vi "getImage.vi"(4 "Streeam":bool, 5 "imageError IN":errorcluster, 6 "Image IN":T1, 7 "errorCamera IN":errorcluster, 8 "hCamera IN":u32) -> (0 "errorImage OUT":errorcluster, 1 "Image OUT":T1, 2 "errorCamera OUT":errorcluster, 3 "hCamera OUT":u32)   [LabVIEW 2010]
uses:
  <vilib>/vision/Image Controls.llb/IMAQ Image.ctl
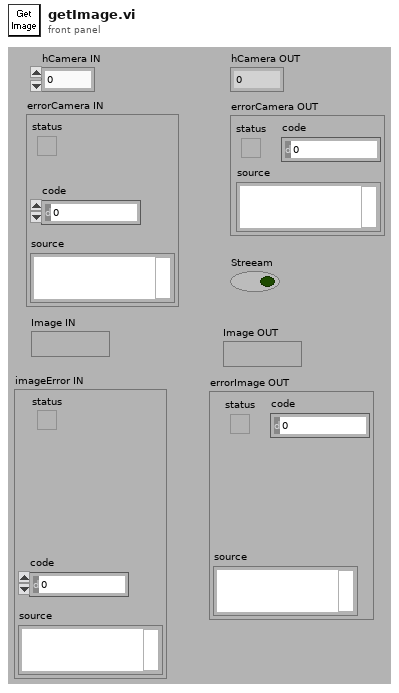
[diagram p1: front panel]
types:
  T1 = typedef "IMAQ Image.ctl" = refnum<image>
  T2 = enum32{"Map Pixel Pointer", "Unmap Pixel Pointer", "Get Pixels Infos"}
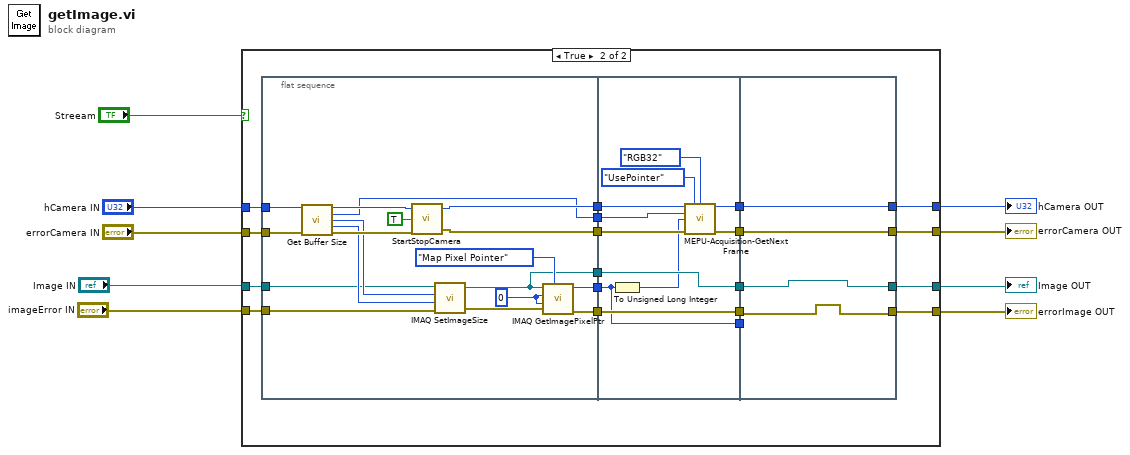
[diagram p0: block diagram]
diagram:
  n1 = case shown="True" "Streeam" {
    tunnel: "hCamera IN" -> [w13 w27]
    tunnel: "errorCamera IN" -> [w12 w26]
    tunnel: "Image IN" -> [w11 w25]
    tunnel: "imageError IN" -> [w10 w24]
    tunnel: [w11 w23] -> w4
    tunnel: [w10 w22] -> w3
    tunnel: [w12 w21] -> w2
    tunnel: [w13 w20] -> w1
    frame False {
    }
    frame True {
      n2 = flat-sequence {
        tunnel: [w48] -> w32
        tunnel: [w47] -> w31
        tunnel: w25 -> [w44]
        tunnel: w24 -> [w43]
        tunnel: w27 -> [w42]
        tunnel: w26 -> [w41]
        tunnel: [w38] -> w30
        tunnel: [w37] -> w29
        tunnel: [w36] -> w28
        tunnel: [w34] -> w19
        tunnel: w32 -> [w61]
        tunnel: w31 -> [w60]
        tunnel: w30 -> [w51]
        tunnel: w29 -> [w54]
        tunnel: w28 -> [w55]
        tunnel: w19 -> [w59]
        tunnel: [w56] -> w18
        tunnel: [w55] -> w17
        tunnel: [w54] -> w16
        tunnel: [w53] -> w15
        tunnel: [w51] -> w14
        tunnel: [w64] -> w21
        tunnel: [w62] -> w22
        tunnel: [w63] -> w23
        tunnel: [w65] -> w20
        tunnel: w18 -> [w65]
        tunnel: w17 -> [w63]
        tunnel: w16 -> [w62]
        tunnel: w15 -> [w64]
        tunnel: w14 -> [_]
        frame #0 {
          w33 = 0 ("Y Coordinate")
          n3 = call "Get Buffer Size.vi"("phCamera IN"=w42, "Error IN"=w41) -> ("phCamera OUT"=w50:u32, "uBufferSize OUT"=w34:u32, "uWidth OUT"=w46:u32, "uHeight OUT"=w45:u32, "Error OUT"=w49:errorcluster)  [unwired: 9 out]
          n4 = call "StartStopCamera.vi"("Error IN"=w49, "Camara ON?"=TRUE, "hCamera IN"=w50) -> ("Error OUT"=w47:errorcluster, "hCamera OUT"=w48:u32)  [unwired: 1 in]
          n5 = call "IMAQ SetImageSize"("error in (no error)"=w43, "Y Resolution"=w45, "X Resolution"=w46, "Image"=w44) -> ("error out"=w40:errorcluster, "Image Out"=w36:T1)  [unwired: 1 in]
          n6 = call "IMAQ GetImagePixelPtr"("Function"=T2."Map Pixel Pointer", "error in (no error)"=w40, "Y Coordinate"=w33, "X Coordinate"=w33, "Image"=w36) -> ("error out"=w37:errorcluster, "Pixel Pointer out"=w38:u64)  [unwired: 1 in, 4 out]
        }
        frame #1 {
          n7 = To Unsigned Long Integer(number=w51) -> (unsigned 32bit integer=w52:u32)
          n8 = call <vilib>:"MEPU-Acquisition-GetNextFrame.vi"("hCamera IN"=w61, "Mode IN"=enum16{"UseArray", "UsePointer"}."UsePointer", "OutputMode IN"=enum16{"Default", "RGB24", "RGB32"}."RGB32", "uBufferSize IN"=w59, "pPixel IN"=w52, "Error IN"=w60) -> ("hCamera OUT"=w56:u32, "Error OUT"=w53:errorcluster)  [unwired: 5 in, 3 out]
        }
        frame #2 {
        }
      }
    }
  }
  "Image OUT" <- w4
  "errorImage OUT" <- w3
  "errorCamera OUT" <- w2
  "hCamera OUT" <- w1
